vi "initVarableList.vi"() -> ()   [LabVIEW 2010]
uses:
  VarableID.ctl
  AmmeterGlobalCostants.vi
panel:
  in  "Array 2":cluster{"CommandCode":string, "VarableID":T1}[](array[cluster])
  out "Numeric":i32
  in  "VarableID":T1
  out "Array":T2(array[cluster])
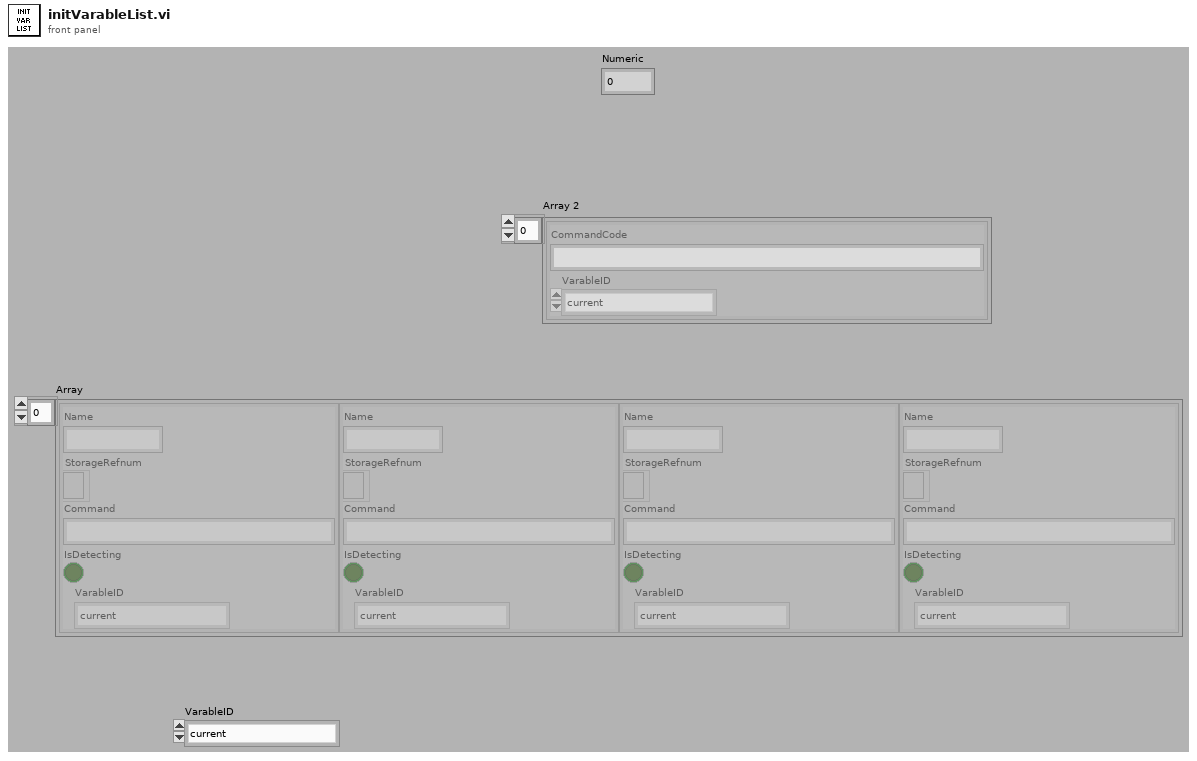
[diagram p1: front panel]
types:
  T1 = typedef "VarableID.ctl" = enum16{"current", "voltage", "power", "PF"}
  T2 = cluster{"Name":string, "StorageRefnum":refnum<file>, "Command":string, "IsDetecting":bool, "VarableID":T1}[]
  T3 = cluster{"Name":string, "StorageRefnum":refnum<file>, "Command":string, "IsDetecting":bool, "VarableID":T1}
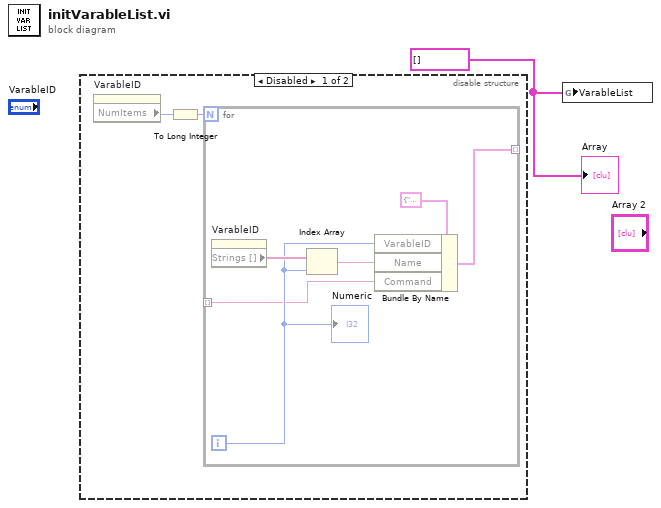
[diagram p0: block diagram]
diagram:
  w1 = T2 []
  n1 = disable-structure shown="Disabled" {
    frame Disabled {
      n2 = property on="VarableID" class="Enum (strict)"() -> ("NumItems"=w2:u32)  [unwired: 2 in, 2 out]
      n3 = To Long Integer(number=w2) -> (32bit integer=w3:i32)
      n4 = for {
        N: w3 -> [_]
        tunnel: [w9] -> _ mode=indexing
        tunnel: _ -> [w4] mode=indexing
        i -> [w5]
        n5 = property on="VarableID" class="Enum (strict)"() -> ("Strings []"=w8:string[])  [unwired: 2 in, 2 out]
        n6 = Index Array(array=w8, index=w5) -> (element=w7:string)
        n7 = Bundle By Name(cluster=T3 {"Name"="", "StorageRefnum"=refnum, "Command"="", "IsDetecting"=FALSE, "VarableID"=enum."current"} ("Varables"), "VarableID"=w5, "Name"=w7, "Command"=w4) -> (w9:T3)
        "Numeric" <- w5
      }
    }
    frame Enabled {
    }
  }
  n8 = global write "AmmeterGlobalCostants.vi" "VarableList"(w1) -> ()
  "Array" <- w1
